vi "并道从文件读取.vi"(1 "并道":enum16{"8192道", "4096道", "2048道", "1024道"}(ring)) -> (0 "波形图":i64[](graph))   [LabVIEW 2014]
uses:
  <vilib>/Utility/file.llb/Read From Spreadsheet File (I64).vi
panel:
  in  "file path (dialog if empty)":path caption="文件路径 （空时为对话框）"
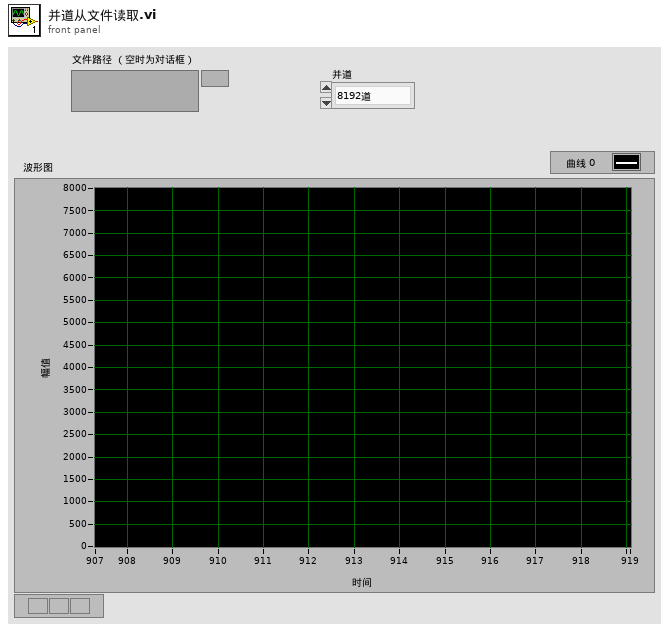
[diagram p1: front panel]
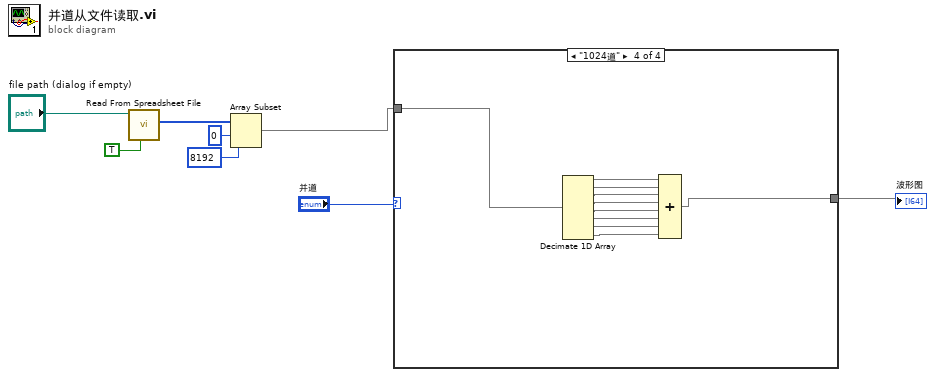
[diagram p0: block diagram]
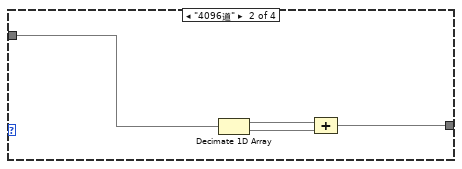
[diagram p3: hidden frame]
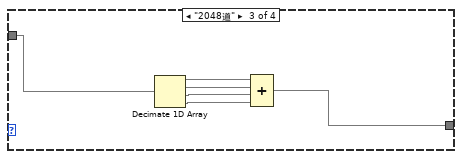
[diagram p4: hidden frame]
diagram:
  n1 = call-poly <vilib>:"Read From Spreadsheet File.vi"("transpose (no:F)"=TRUE, "file path (dialog if empty)"="file path (dialog if empty)") -> ("first row"=w4:i64[])  [unwired: 5 in, 4 out]
  n2 = Array Subset(array=w4, index=0 ("索引"), length=8192 ("长度")) -> (w1:i64[])
  n3 = case shown="\"1024道\"" "并道" {
    tunnel: w1 -> [w9 w13 w15 w21]
    tunnel: [w9 w10 w14 w20] -> w7
    frame "8192道", Default {
    }
    frame "4096道" {
      n4 = Decimate 1D Array(w13) -> (w12:i64[], w11:i64[])
      n5 = Compound Arithmetic op=ADD(w12, w11) -> (w10:i64[])
    }
    frame "2048道" {
      n6 = Decimate 1D Array(w15) -> (w19:i64[], w18:i64[], w17:i64[], w16:i64[])
      n7 = Compound Arithmetic op=ADD(w19, w18, w17, w16) -> (w14:i64[])
    }
    frame "1024道" {
      n8 = Decimate 1D Array(w21) -> (w29:i64[], w28:i64[], w27:i64[], w26:i64[], w25:i64[], w24:i64[], w23:i64[], w22:i64[])
      n9 = Compound Arithmetic op=ADD(w29, w28, w27, w26, w25, w24, w23, w22) -> (w20:i64[])
    }
  }
  "波形图" <- w7
